vi "EVB Calculate connector repeatability.vi"() -> ()   [LabVIEW 2020]
uses:
  <vilib>/addons/HF Network Analysis/Support VIs/Read SnP File (SnP).vi
  <vilib>/addons/HF Network Analysis/NI_HFNetworkAnalysis.lvlib
panel:
  out "XY Graph":cluster{dbl[], dbl[]}(graph)
  out "Array 2":i32[][](array[numeric])
  out "max index(es)":i32[](array[numeric])
  out "XY Graph 2":cluster{dbl[], dbl[]}[](graph)
  out "x*y":dbl[][](array[numeric])
  out "Array":cdb[][](array[numeric])
  out "S-parameters":cdb[][](array[numeric])
  out "Frequencies (Hz)":dbl[](array[numeric])
  in  "SnP File Path":path
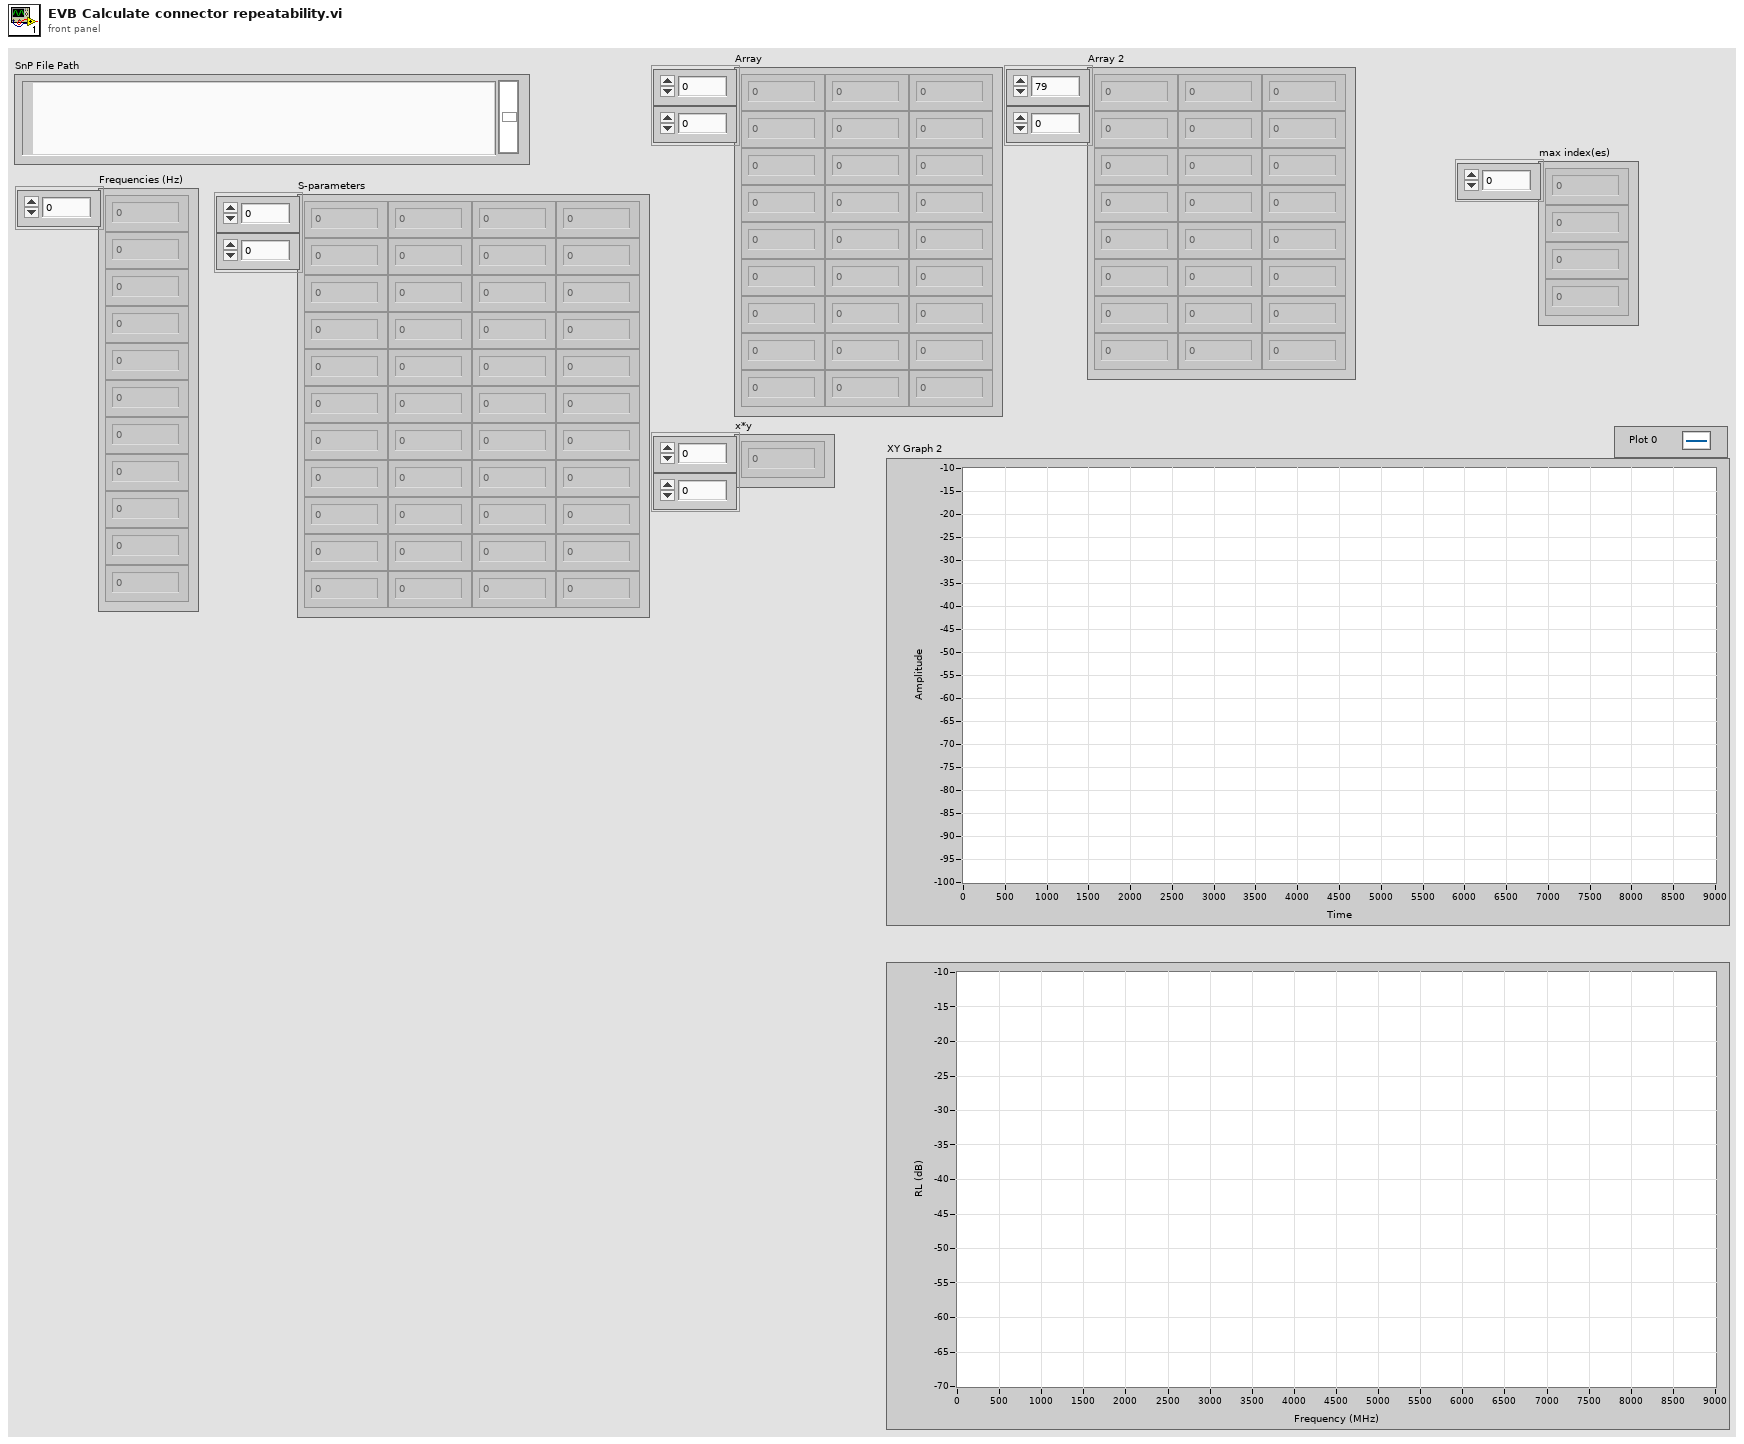
[diagram p1: front panel]
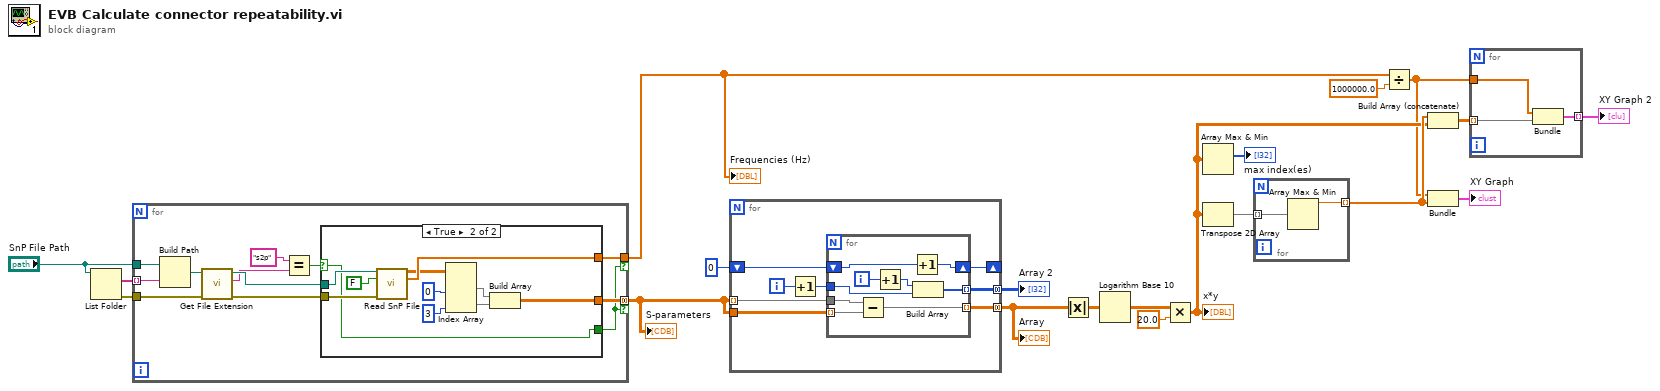
[diagram p0: block diagram]
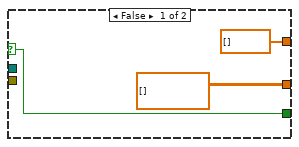
[diagram p2: hidden frame]
diagram:
  n1 = List Folder(path="SnP File Path") -> (filenames=w19:string[], error out=w20:errorcluster)  [unwired: 3 in, 2 out]
  n2 = for {
    tunnel: w20 -> [w31]
    tunnel: w19 -> [w30] mode=indexing
    tunnel: "SnP File Path" -> [w29]
    tunnel: [w23] -> w7 if=w21
    tunnel: [w22] -> w17 mode=concatenating if=w21
    n3 = Build Path(base path=w29, name or relative path=w30) -> (appended path=w32:path)
    n4 = call <vilib>:"Get File Extension.vi"("error in (no error)"=w31, "file"=w32) -> ("error out"=w28:errorcluster, "lowercase file extension"=w25:string, "dup file"=w27:path)  [unwired: 5 in, 2 out]
    n5 = Equal?(x="s2p" ("regular expression"), y=w25) -> (x = y?=w24:bool)
    n6 = case shown="True" w24 {
      selector: w24 -> [w34 w42]
      tunnel: w28 -> [_ w45]
      tunnel: w27 -> [_ w44]
      tunnel: [dbl[] [] ("Frequencies (Hz)") w43] -> w23
      tunnel: [cdb[][] [] ("S-parameters") w36] -> w22
      tunnel: [w34 w42] -> w21
      frame False {
      }
      frame True {
        n7 = call-poly <vilib>:"Read SnP File.vi"("SnP File Path"=w44, "Swap Ports (False)"=FALSE, "Error In"=w45) -> ("S-parameters"=w41:cdb[][], "Frequencies (Hz)"=w43:dbl[])  [unwired: 9 in, 2 out]
        n8 = Index Array(array=w41, index (col) #1=0 ("disabled index (col)"), index (col) #2=3 ("index (col)")) -> (element #1=w38:cdb[], element #2=w37:cdb[])  [unwired: 2 in]
        n9 = Build Array(w38, w37) -> (w36:cdb[][])
      }
    }
  }
  "Frequencies (Hz)" <- w7
  "S-parameters" <- w17
  n10 = for {
    tunnel: w17 -> [w53] mode=indexing
    tunnel: w17 -> [w54]
    tunnel: [w52] -> w10 mode=concatenating
    shift-right: [w51] -> _
    shift-left: 0 -> [w50]
    tunnel: [w49] -> w11 mode=concatenating
    i -> [w48]
    n11 = Increment(x=w48) -> (x+1=w47:i32)
    n12 = for {
      tunnel: w54 -> [w62] mode=indexing
      tunnel: w53 -> [w63]
      tunnel: [w61] -> w52 mode=indexing
      shift-right: [w60] -> w51
      shift-left: w50 -> [w59]
      tunnel: w47 -> [w58]
      tunnel: [w57] -> w49 mode=indexing
      i -> [w56]
      n13 = Subtract(x=w63, y=w62) -> (x-y=w61:cdb[])
      n14 = Increment(x=w56) -> (x+1=w55:i32)
      n15 = Increment(x=w59) -> (x+1=w60:i32)
      n16 = Build Array(w55, w58) -> (w57:i32[])
    }
  }
  "Array" <- w10
  "Array 2" <- w11
  n17 = Absolute Value(x=w10) -> (abs(x)=w15:dbl[][])
  n18 = Logarithm Base 10(1:w15) -> (0:w16:dbl[][])
  n19 = Multiply(x=w16, y=20.0) -> (x*y=w4:dbl[][])
  "x*y" <- w4
  n20 = Array Max & Min(array=w4) -> (max index (indices)=→"max index(es)":i32[])  [unwired: 3 out]
  n21 = Transpose 2D Array(2D array=w4) -> (transposed array=w9:dbl[][])
  n22 = for {
    tunnel: w9 -> [w65] mode=indexing
    tunnel: [w64] -> w5 mode=indexing
    n23 = Array Max & Min(array=w65) -> (max value=w64:dbl)  [unwired: 3 out]
  }
  n24 = Divide(x=w7, y=1000000.0) -> (x/y=w2:dbl[])
  n25 = Build Array (concatenate)(w5, w4) -> (w3:dbl[][])
  n26 = Bundle(w2, w5) -> (→"XY Graph":cluster{dbl[], dbl[]})  [unwired: 1 in]
  n27 = for {
    tunnel: w3 -> [w67] mode=indexing
    tunnel: w2 -> [w68]
    tunnel: [w66] -> w1 mode=indexing
    n28 = Bundle(w68, w67) -> (w66:cluster{dbl[], dbl[]})  [unwired: 1 in]
  }
  "XY Graph 2" <- w1
